vi "GDFsaveDataToXML.vi"(0 "GDFv1.x.lvclass":refnum<class "GDFv1.x.lvclass">, 1 "Array of indexes":i32[](array[numeric]), 6 "XML file path":path, 7 "Duration":dbl) -> (14 "output cluster":refnum<class "GDFv1.x.lvclass">, 19 "error out":errorcluster)   [LabVIEW 2016, in "GDF File Reader.lvlib" / "GDFv1.x.lvclass"]
uses:
  GDFv1.x.lvclass
  _XML_EEG_File_Parser/_vlib/XML_EEG_Header.ctl
  _XML_EEG_File_Parser/_vlib/XML_EEG_Dataset.ctl
  _XML_EEG_File_Parser/_vlib/XML_EEG_File.lvclass
  GDFv1.x.lvclass/GDFv1.x.ctl
  <vilib>/Waveform/WDTOps.llb/WDT Get Waveform Subset DBL.vi
  _XML_EEG_File_Parser/XML_EEG_File_Parser.lvlib
panel:
  # "This VI is a part of BCI Design library, http://www.ru-bci.org \nCopyright © 2020, Sotnikov Peter, All rights reserved. License: CC BY-NC 4.0"
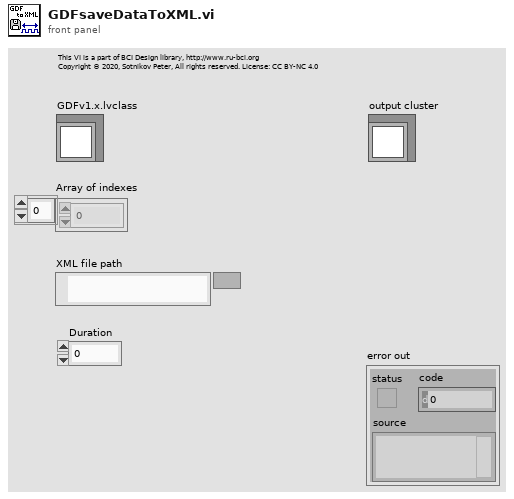
[diagram p1: front panel]
types:
  T1 = typedef "XML_EEG_File_Parser.lvlib/XML_EEG_Dataset.ctl" = cluster{"Attributes":cluster{"NumberOfSamples":i32, "StartDateTime":timestamp}, "Body":cluster{"MarkerValue":string, "Channels":waveform(dbl)[]}}
  T2 = typedef "XML_EEG_File_Parser.lvlib/XML_EEG_Header.ctl" = cluster{"Attributes":cluster{"ChannelDataType":string, "NumberOfChannels":i32, "SampleRateHz":dbl, "MarkerChannel":i32}, "Body":cluster{"PatientSpecificData":string, "NumberOfDatasets":i32, "Channels":string[]}}
  T3 = typedef "GDF File Reader.lvlib/EventDataType.ctl" = cluster{"Position (in samples)":u32, "EventType":string, "Channel":u16, "Duration (in samples)":u32}
  T4 = typedef "GDF File Reader.lvlib/GdfHeader1.ctl" = cluster{"Version identificator":string, "Patient identificator":string, "Recording identificator":string, "StartDateTime":timestamp, "Header record length":i64, "Equipment Provider":u64, "Laboratory":u64, "Technician":u64, "Number of data records":i64, "Duration of a data record":cluster{"Numerator":u32, "Denominator":u32}, "Number of signals":u32}
  T5 = typedef "GDF File Reader.lvlib/GdfHeader2.ctl" = cluster{"Channel labels":string[], "Transduser types":string[], "Physical dimensions":string[], "Physical lows":dbl[], "Physical highs":dbl[], "Digital lows":dbl[], "Digital highs":dbl[], "Channels Pre-filtering":string[], "Number of samples":u32[], "Channel types":u32[], "Addons":string[]}
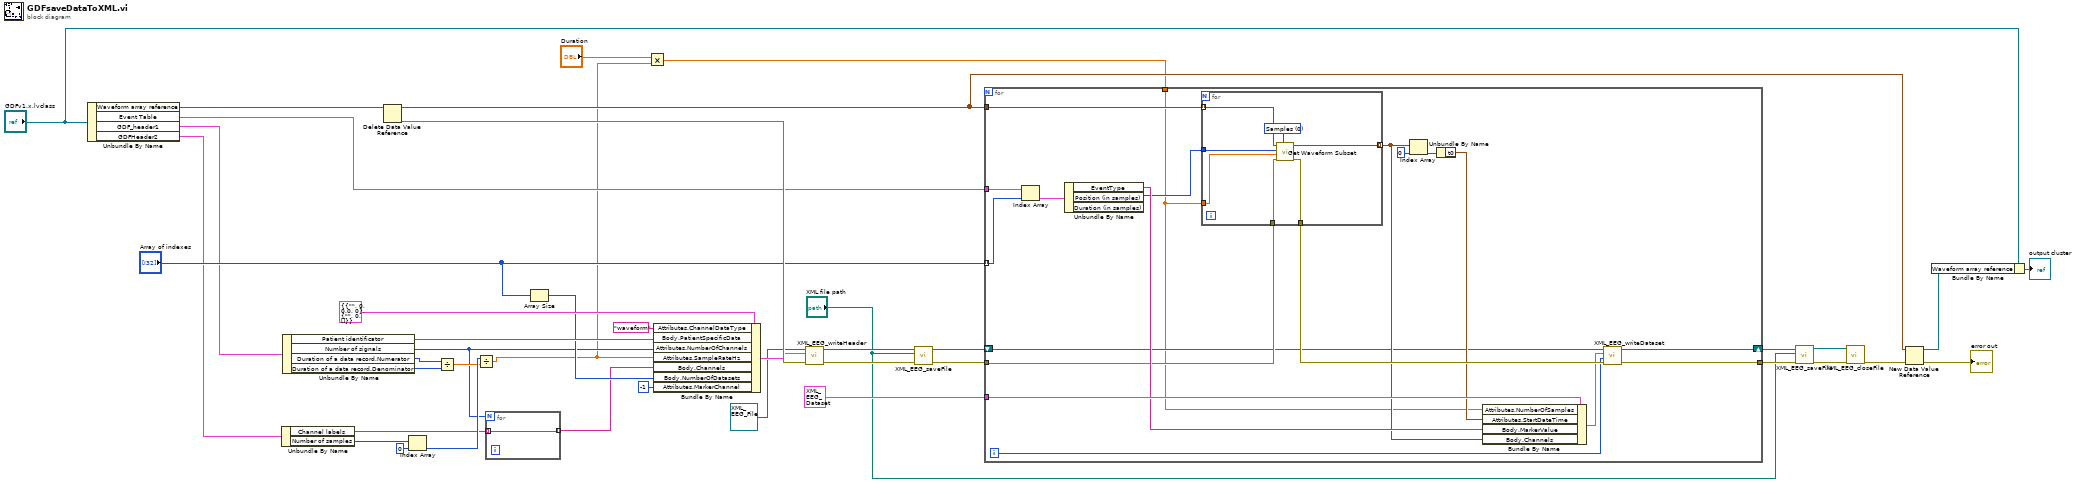
[diagram p0: block diagram]
diagram:
  n1 = Unbundle By Name("GDFv1.x.lvclass") -> ("Waveform array reference"=w26:refnum<data-value>, "Event Table"=w25:T3[], "GDF_header1"=w24:T4, "GDFHeader2"=w23:T5)
  n2 = Unbundle By Name(w23) -> ("Channel labels"=w6:string[], "Number of samples"=w41:u32[])
  n3 = Unbundle By Name(w24) -> ("Patient identificator"=w35:string, "Number of signals"=w4:u32, "Duration of a data record.Numerator"=w39:u32, "Duration of a data record.Denominator"=w38:u32)
  n4 = Delete Data Value Reference(data value reference=w26) -> (data value=w28:waveform(dbl)[], error out=w34:errorcluster)  [unwired: 1 in]
  n5 = Index Array(array=w41, index=0) -> (element=w32:u32)
  n6 = Divide(x=w39, y=w38) -> (x/y=w31:dbl)
  n7 = Divide(x=w32, y=w31) -> (x/y=w3:dbl)
  n8 = for {
    N: w4 -> [_]
    tunnel: w6 -> [w42] mode=indexing
    tunnel: [w42] -> w5 mode=indexing
  }
  n9 = Array Size(array="Array of indexes") -> (size(s)=w30:i32)
  n10 = Multiply(x="Duration", y=w3) -> (x*y=w2:dbl)
  n11 = Bundle By Name(cluster=T2 {"Attributes"={"ChannelDataType"="", "NumberOfChannels"=0, "SampleRateHz"=0.0, "MarkerChannel"=0}, "Body"={"PatientSpecificData"="", "NumberOfDatasets"=0, "Channels"=[]}} ("XML_Header"), "Attributes.ChannelDataType"="waveform", "Body.PatientSpecificData"=w35, "Attributes.NumberOfChannels"=w4, "Attributes.SampleRateHz"=w3, "Body.Channels"=w5, "Body.NumberOfDatasets"=w30, "Attributes.MarkerChannel"=-1) -> (w18:T2)
  n12 = call "XML_EEG_writeHeader.vi"("error in (no error)"=w34, "XML_Header"=w18, "XML_EEG_File in"=refnum<class "XML_EEG_File.lvclass"> refnum ("XML_EEG_File_Parser.lvlib:XML_EEG_File.lvclass")) -> ("error out"=w11:errorcluster, "XML_EEG_File out"=w10:refnum<class "XML_EEG_File.lvclass">)  [unwired: 6 in, 1 out]
  n13 = call "XML_EEG_saveFile.vi"("error in (no error)"=w11, "XML file path"="XML file path", "XML_EEG_File in"=w10) -> ("error out"=w8:errorcluster, "XML_EEG_File out"=w7:refnum<class "XML_EEG_File.lvclass">)  [unwired: 7 in]
  n14 = for {
    tunnel: "Array of indexes" -> [w45] mode=indexing
    tunnel: w25 -> [w61]
    tunnel: w28 -> [w58]
    tunnel: w8 -> [w49]
    tunnel: T1 {"Attributes"={"NumberOfSamples"=0, "StartDateTime"=timestamp(0 s since 1904-01-01)}, "Body"={"MarkerValue"="", "Channels"=[]}} ("XML_Dataset") -> [w59]
    tunnel: [w48] -> w16
    shift-right: [w47] -> w15
    shift-left: w7 -> [w46]
    tunnel: w2 -> [w43]
    i -> [w50]
    n15 = Index Array(array=w61, index=w45) -> (element=w60:T3)
    n16 = Unbundle By Name(w60) -> ("EventType"=w56:string, "Position (in samples)"=w44:u32)  [unwired: 1 out]
    n17 = for {
      tunnel: w58 -> [w68] mode=indexing
      tunnel: w49 -> [w66]
      tunnel: w44 -> [w65]
      tunnel: [w64] -> w57
      tunnel: [w63] -> w55 mode=indexing
      tunnel: w43 -> [w62]
      w67 = u16 0 items=["Samples", "Relative Time"] ("start/duration format")
      n18 = call-poly <vilib>:"Get Waveform Subset.vi"("start/duration format"=w67, "error in (no error)"=w66, "duration"=w62, "start samples/time"=w65, "waveform in"=w68) -> ("error out"=w64:errorcluster, "waveform out"=w63:waveform(dbl))  [unwired: 1 in, 2 out]
    }
    n19 = Index Array(array=w55, index=0) -> (element=w53:waveform(dbl))
    n20 = Unbundle By Name(w53) -> ("t0"=w52:timestamp)
    n21 = Bundle By Name(cluster=w59, "Attributes.NumberOfSamples"=w43, "Attributes.StartDateTime"=w52, "Body.MarkerValue"=w56, "Body.Channels"=w55) -> (w51:T1)
    n22 = call "XML_EEG_writeDataset.vi"("error in (no error)"=w57, "DatasetNumber"=w50, "XML_Dataset"=w51, "XML_EEG_File in"=w46) -> ("error out"=w48:errorcluster, "XML_EEG_File out"=w47:refnum<class "XML_EEG_File.lvclass">)  [unwired: 5 in, 1 out]
  }
  n23 = call "XML_EEG_saveFile.vi"("error in (no error)"=w16, "XML file path"="XML file path", "XML_EEG_File in"=w15) -> ("error out"=w14:errorcluster, "XML_EEG_File out"=w13:refnum<class "XML_EEG_File.lvclass">)  [unwired: 7 in]
  n24 = call "XML_EEG_closeFile.vi"("error in (no error)"=w14, "XML_EEG_File.lvclass"=w13) -> ("error out"=w12:errorcluster)  [unwired: 9 in]
  n25 = New Data Value Reference(data value=w28, error in=w12) -> (data value reference=w21:refnum<data-value>, error out=→"error out":errorcluster)
  n26 = Bundle By Name(cluster="GDFv1.x.lvclass", "Waveform array reference"=w21) -> (→"output cluster":refnum<class "GDFv1.x.lvclass">)
